vi "DevB.Set Frequency.vi"(8 "error in (no error)":errorcluster, 10 "Frequency":i32, 11 "DevB Session in":T1) -> (0 "error out":errorcluster, 3 "DevB Session out":T1)   [LabVIEW 2018]
uses:
  typedefs/DevB.Session.ctl
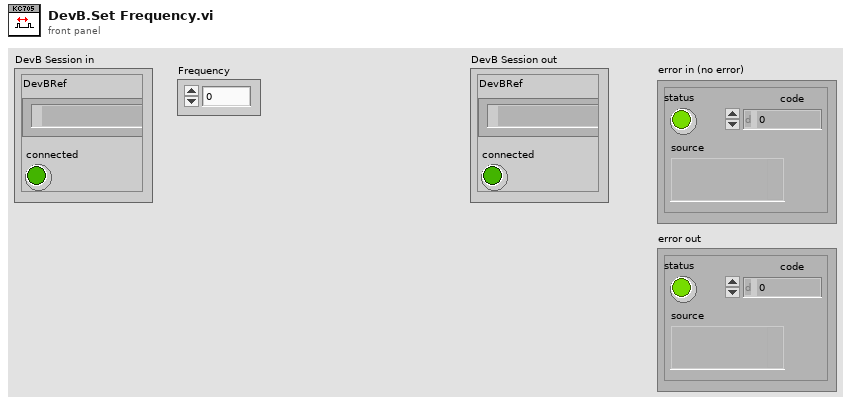
[diagram p1: front panel]
types:
  T1 = typedef "DevB.Session.ctl" = cluster{"DevBRef":refnum<visa-resource-name>, "connected":bool}
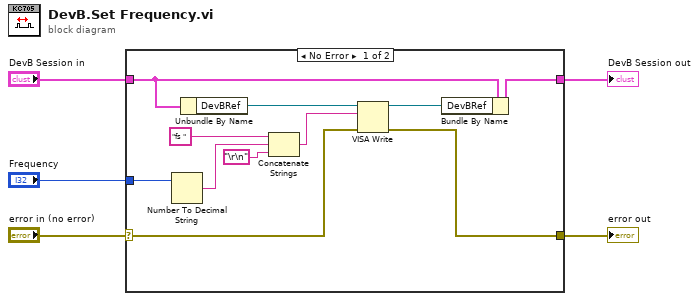
[diagram p0: block diagram]
diagram:
  n1 = case shown="No Error" "error in (no error)" {
    selector: "error in (no error)" -> [w13 w18]
    tunnel: "DevB Session in" -> [w15 w17]
    tunnel: [w12 w18] -> w3
    tunnel: [w11 w17] -> w2
    tunnel: "Frequency" -> [w7 _]
    frame No Error {
      n2 = Number To Decimal String(number=w7) -> (decimal integer string=w9:string)  [unwired: 1 in]
      n3 = Unbundle By Name(w15) -> ("DevBRef"=w16:refnum<visa-resource-name>)
      n4 = Concatenate Strings("fs ", w9, "\r\n") -> (w8:string)
      n5 = VISA Write(VISA resource name=w16, write buffer=w8, error in (no error)=w13) -> (VISA resource name out=w14:refnum<visa-resource-name>, error out=w12:errorcluster)  [unwired: 1 out]
      n6 = Bundle By Name(cluster=w15, "DevBRef"=w14) -> (w11:T1)
    }
    frame Error {
    }
  }
  "DevB Session out" <- w2
  "error out" <- w3
